vi "CheckDataPackets.vi"() -> ()   [LabVIEW 2012]
panel:
  out "x = y?":bool=TRUE
  out "unsigned byte array 2":u8[](array[numeric])=[0, 115, 0, 3, 0, 18, 5, 61, 0, 0, 0, 1, 5, 61, 0, 1, 0, 0, 5, 61, 0, 2, 0, 1, 5, 61, 0, 3, 0, 0, 5, 61, 0, 4, 247, 3, 5, 61, 0, 5, 255, 2, 5, 42, 0, 5, 255, 4, 5, 61, 0, 1, 255, 5, 5, 61, 0, 5, 255, 0, 5, 43, 0, 5, 255, 1, 5, 61, 0, 0, 255, 5, 5, 61, 0, 5, 255, 2, 5, 42, 0, 5, 0, 2, 5, 61, 0, 2, 255, 5, 5, 43, 0, 3, 0, 1, 8, 73, 60, 255, 3, 0, 14, 0, 24] format="%.0x"
  out "Array 2":u8[][](array[numeric])=[[5, 61, 0, 0, 0, 1, 0, 0, 0], [5, 61, 0, 1, 0, 0, 0, 0, 0], [5, 61, 0, 2, 0, 1, 0, 0, 0], [5, 61, 0, 3, 0, 0, 0, 0, 0], [5, 61, 0, 4, 247, 3, 0, 0, 0], [5, 61, 0, 5, 255, 2, 0, 0, 0], [5, 42, 0, 5, 255, 4, 0, 0, 0], [5, 61, 0, 1, 255, 5, 0, 0, 0], [5, 61, 0, 5, 255, 0, 0, 0, 0], [5, 43, 0, 5, 255, 1, 0, 0, 0], [5, 61, 0, 0, 255, 5, 0, 0, 0], [5, 61, 0, 5, 255, 2, 0, 0, 0], [5, 42, 0, 5, 0, 2, 0, 0, 0], [5, 61, 0, 2, 255, 5, 0, 0, 0], [5, 43, 0, 3, 0, 1, 0, 0, 0], [8, 73, 60, 255, 3, 0, 14, 0, 24]]
  out "Array":u8[][](array[numeric])=[[5, 61, 0, 0, 0, 1, 0, 0, 0], [5, 61, 0, 1, 0, 0, 0, 0, 0], [5, 61, 0, 2, 0, 1, 0, 0, 0], [5, 61, 0, 3, 0, 0, 0, 0, 0], [5, 61, 0, 4, 247, 3, 0, 0, 0], [5, 61, 0, 5, 255, 2, 0, 0, 0], [5, 42, 0, 5, 255, 4, 0, 0, 0], [5, 61, 0, 1, 255, 5, 0, 0, 0], [5, 61, 0, 5, 255, 0, 0, 0, 0], [5, 43, 0, 5, 255, 1, 0, 0, 0], [5, 61, 0, 0, 255, 5, 0, 0, 0], [5, 61, 0, 5, 255, 2, 0, 0, 0], [5, 42, 0, 5, 0, 2, 0, 0, 0], [5, 61, 0, 2, 255, 5, 0, 0, 0], [5, 43, 0, 3, 0, 1, 0, 0, 0], [8, 73, 60, 255, 3, 0, 14, 0, 24]]
  out "unsigned byte array":u8[](array[numeric])=[5, 61, 0, 0, 0, 1, 5, 61, 0, 1, 0, 0, 5, 61, 0, 2, 0, 1, 5, 61, 0, 3, 0, 0, 5, 61, 0, 4, 247, 3, 5, 61, 0, 5, 255, 2, 5, 42, 0, 5, 255, 4, 5, 61, 0, 1, 255, 5, 5, 61, 0, 5, 255, 0, 5, 43, 0, 5, 255, 1, 5, 61, 0, 0, 255, 5, 5, 61, 0, 5, 255, 2, 5, 42, 0, 5, 0, 2, 5, 61, 0, 2, 255, 5, 5, 43, 0, 3, 0, 1, 8, 73, 60, 255, 3, 0, 14, 0, 24]
  in  "resulting string":string="\u0005=\u0000\u0000\u0000\u0001\u0005=\u0000\u0001\u0000\u0000\u0005=\u0000\u0002\u0000\u0001\u0005=\u0000\u0003\u0000\u0000\u0005=\u0000\u0004÷\u0003\u0005=\u0000\u0005ÿ\u0002\u0005*\u0000\u0005ÿ\u0004\u0005=\u0000\u0001ÿ\u0005\u0005=\u0000\u0005ÿ\u0000\u0005+\u0000\u0005ÿ\u0001\u0005=\u0000\u0000ÿ\u0005\u0005=\u0000\u0005ÿ\u0002\u0005*\u0000\u0005\u0000\u0002\u0005=\u0000\u0002ÿ\u0005\u0005+\u0000\u0003\u0000\u0001\bI<ÿ\u0003\u0000\u000e\u0000\u0018"
  in  "read buffer":string="R:[ 115 0 3 0 18 5 61 0 0 0 1 5 61 0 1 0 0 5 61 0 2 0 1 5 61 0 3 0 0 5 61 0 4 247 3 5 61 0 5 255 2 5 42 0 5 255 4 5 61 0 1 255 5 5 61 0 5 255 0 5 43 0 5 255 1 5 61 0 0 255 5 5 61 0 5 255 2 5 42 0 5 0 2 5 61 0 2 255 5 5 43 0 3 0 1 8 73 60 255 3 0 14 0 24] "
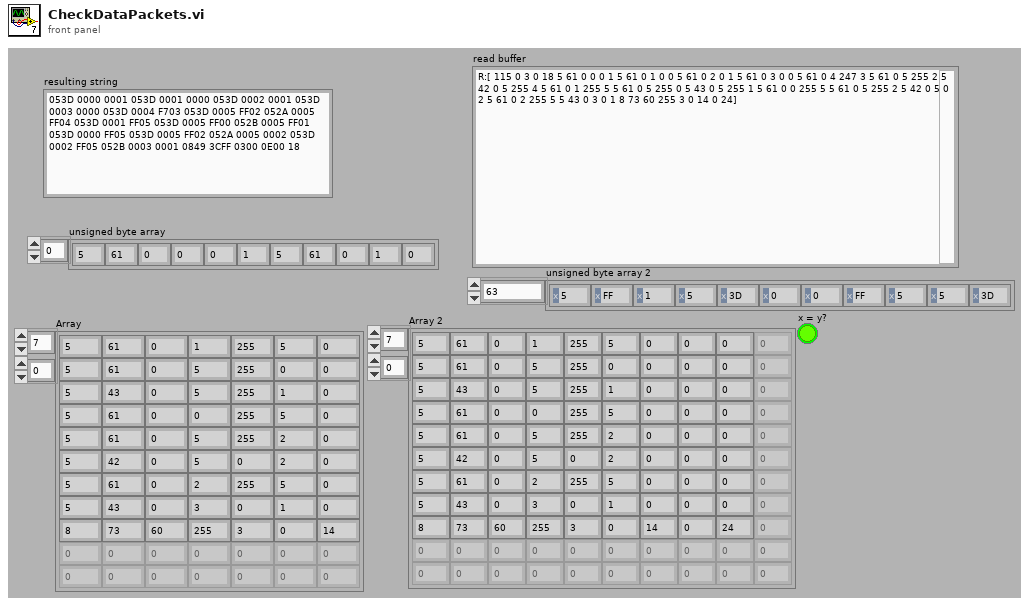
[diagram p1: front panel]
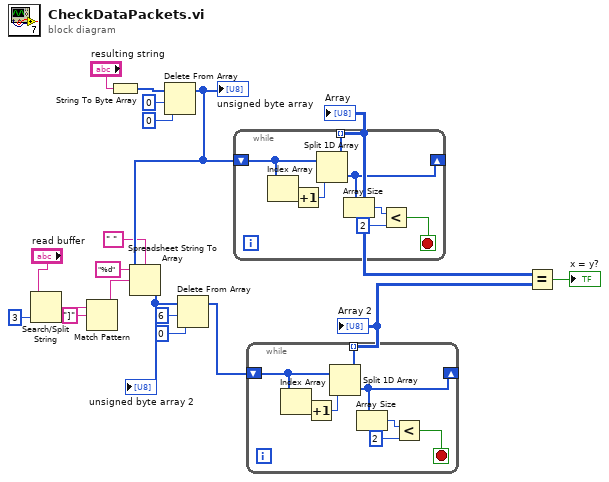
[diagram p0: block diagram]
diagram:
  n1 = Search/Split String(string="read buffer", offset (0)=3) -> (match + rest of string=w10:string)  [unwired: 1 in, 2 out]
  n2 = Match Pattern(string=w10, regular expression="]") -> (before substring=w9:string)  [unwired: 1 in, 3 out]
  n3 = String To Byte Array(string="resulting string") -> (unsigned byte array=w18:u8[])
  n4 = Delete From Array(array=w18, length=0, index=0) -> (array with subset deleted=w8:u8[])  [unwired: 1 out]
  "unsigned byte array" <- w8
  n5 = Spreadsheet String To Array(delimiter (Tab)=" ", format string="%d", spreadsheet string=w9, array type (2D Dbl)=w8) -> (array=w4:u8[])
  "unsigned byte array 2" <- w4
  n6 = Delete From Array(array=w4, length=6, index=0) -> (array with subset deleted=w15:u8[])  [unwired: 1 out]
  n7 = while {
    shift-right: [w25] -> _
    shift-left: w8 -> [w27]
    tunnel: [w21] -> w3 mode=indexing
    stop <- w22 stop-if-true
    n8 = Index Array(array=w27) -> (element=w26:u8)  [unwired: 1 in]
    n9 = Increment(x=w26) -> (x+1=w20:u8)
    n10 = Split 1D Array(array=w27, index=w20) -> (first subarray=w21:u8[], second subarray=w25:u8[])
    n11 = Array Size(array=w25) -> (size(s)=w24:i32)
    n12 = Less?(x=w24, y=2) -> (x < y?=w22:bool)
  }
  "Array" <- w3
  n13 = while {
    shift-right: [w33] -> _
    shift-left: w15 -> [w35]
    tunnel: [w29] -> w2 mode=indexing
    stop <- w30 stop-if-true
    n14 = Index Array(array=w35) -> (element=w34:u8)  [unwired: 1 in]
    n15 = Increment(x=w34) -> (x+1=w28:u8)
    n16 = Split 1D Array(array=w35, index=w28) -> (first subarray=w29:u8[], second subarray=w33:u8[])
    n17 = Array Size(array=w33) -> (size(s)=w32:i32)
    n18 = Less?(x=w32, y=2) -> (x < y?=w30:bool)
  }
  "Array 2" <- w2
  n19 = Equal?(x=w3, y=w2) -> (x = y?=→"x = y?":bool)
